vi "start waveform.vi"(4 "length":u16, 5 "time":dbl, 6 "trig_level":u32, 7 "trig_mask":u32, 8 "error in (no error)":errorcluster, 9 "dec_ratio":u16, 10 "mode":u16, 11 "identifier":string) -> (0 "error out":errorcluster, 3 "function return":u32)   [LabVIEW 2015, in "XGL_DPP.lvlib"]
doc: "EXTERN DECLSPEC uint32_t CALL_CONV start_waveform(const char * identifier,\n uint16_t mode,\n uint16_t dec_ratio,\n uint32_t trig_mask,\n uint32_t trig_level,\n const double time,\n uint16_t length);"
uses:
  XGL_DPP.lvlib
  XGL_DPP.dll
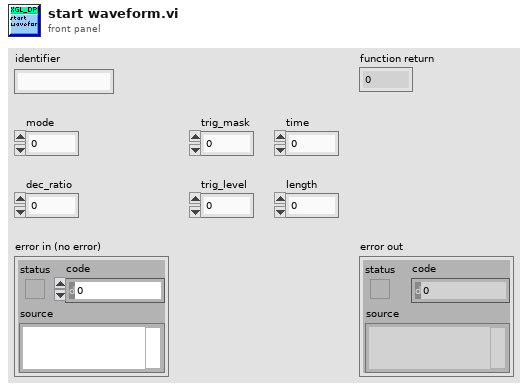
[diagram p1: front panel]
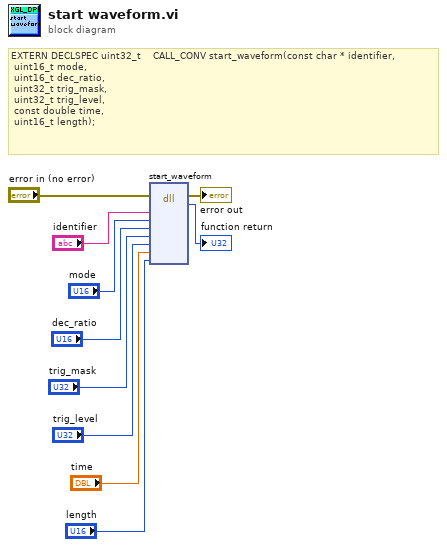
[diagram p0: block diagram]
diagram:
  # "EXTERN DECLSPEC uint32_t    CALL_CONV start_waveform(const char * identifier,\n\tuint16_t mode,\n\tuint16_t dec_ratio,\n\tuint32_t trig_mask,\n\tuint32_t trig_level,\n\tconst double time,\n\tuint16_t length);"
  n1 = dll-call lib="D:/Users/XRF/Desktop/Scanning Software_Demokritos_2015_v7/libs/Vis_2/XGL_DPP.*" fn="start_waveform"(error in="error in (no error)", "identifier"="identifier", "mode"="mode", "dec_ratio"="dec_ratio", "trig_mask"="trig_mask", "trig_level"="trig_level", "time"="time", "length"="length") -> (error out=→"error out":errorcluster, →"function return":u32)  [unwired: 9 in, 1 out]
